vi "Compass on GIC parallel 2.vi"(11 "GIC Input 2":T1={"     Use ?\nOff       On"=[FALSE, TRUE, FALSE, TRUE], "Mode:"=FALSE, "Extra Port"="", "Hokuyo Port"="COM7", "Tx Prop  Port"="COM6", "Compass Port"="", "GPS Port"="", "Num of WPs"=0, "WP Lats and Longs"={"WP Lats"=[], "WP Longs"=[]}, "Obst Lats and Longs"={"Obst Lats"=[], "Obst Longs"=[]}, "Parameters"=[], "GPS Data"=[], "Compass"=0.0, "LMS Vector"=[], "Vision Vector"=[], "Direction Cmd"=0.0, "Speed Cmd"=0.0, "WP Vector"=[], "WP Number"=0, "Extra"=0, "SW Map"=[], "Path Cluster"={"Path x node"=[], "Path y node"=[]}, "Sim Course"=[]} {"Obst Lats and Longs"."Obst Longs" format="%#_8g"; "Obst Lats and Longs"."Obst Lats" format="%#_8g"}) -> ()   [LabVIEW 2014]
uses:
  Global_vars.vi
panel:
  out "compass out":dbl
  # "Compass on GIC parallel 2"
  # "Compass on New GIC A"
  # "Input:"
  # "Output:"
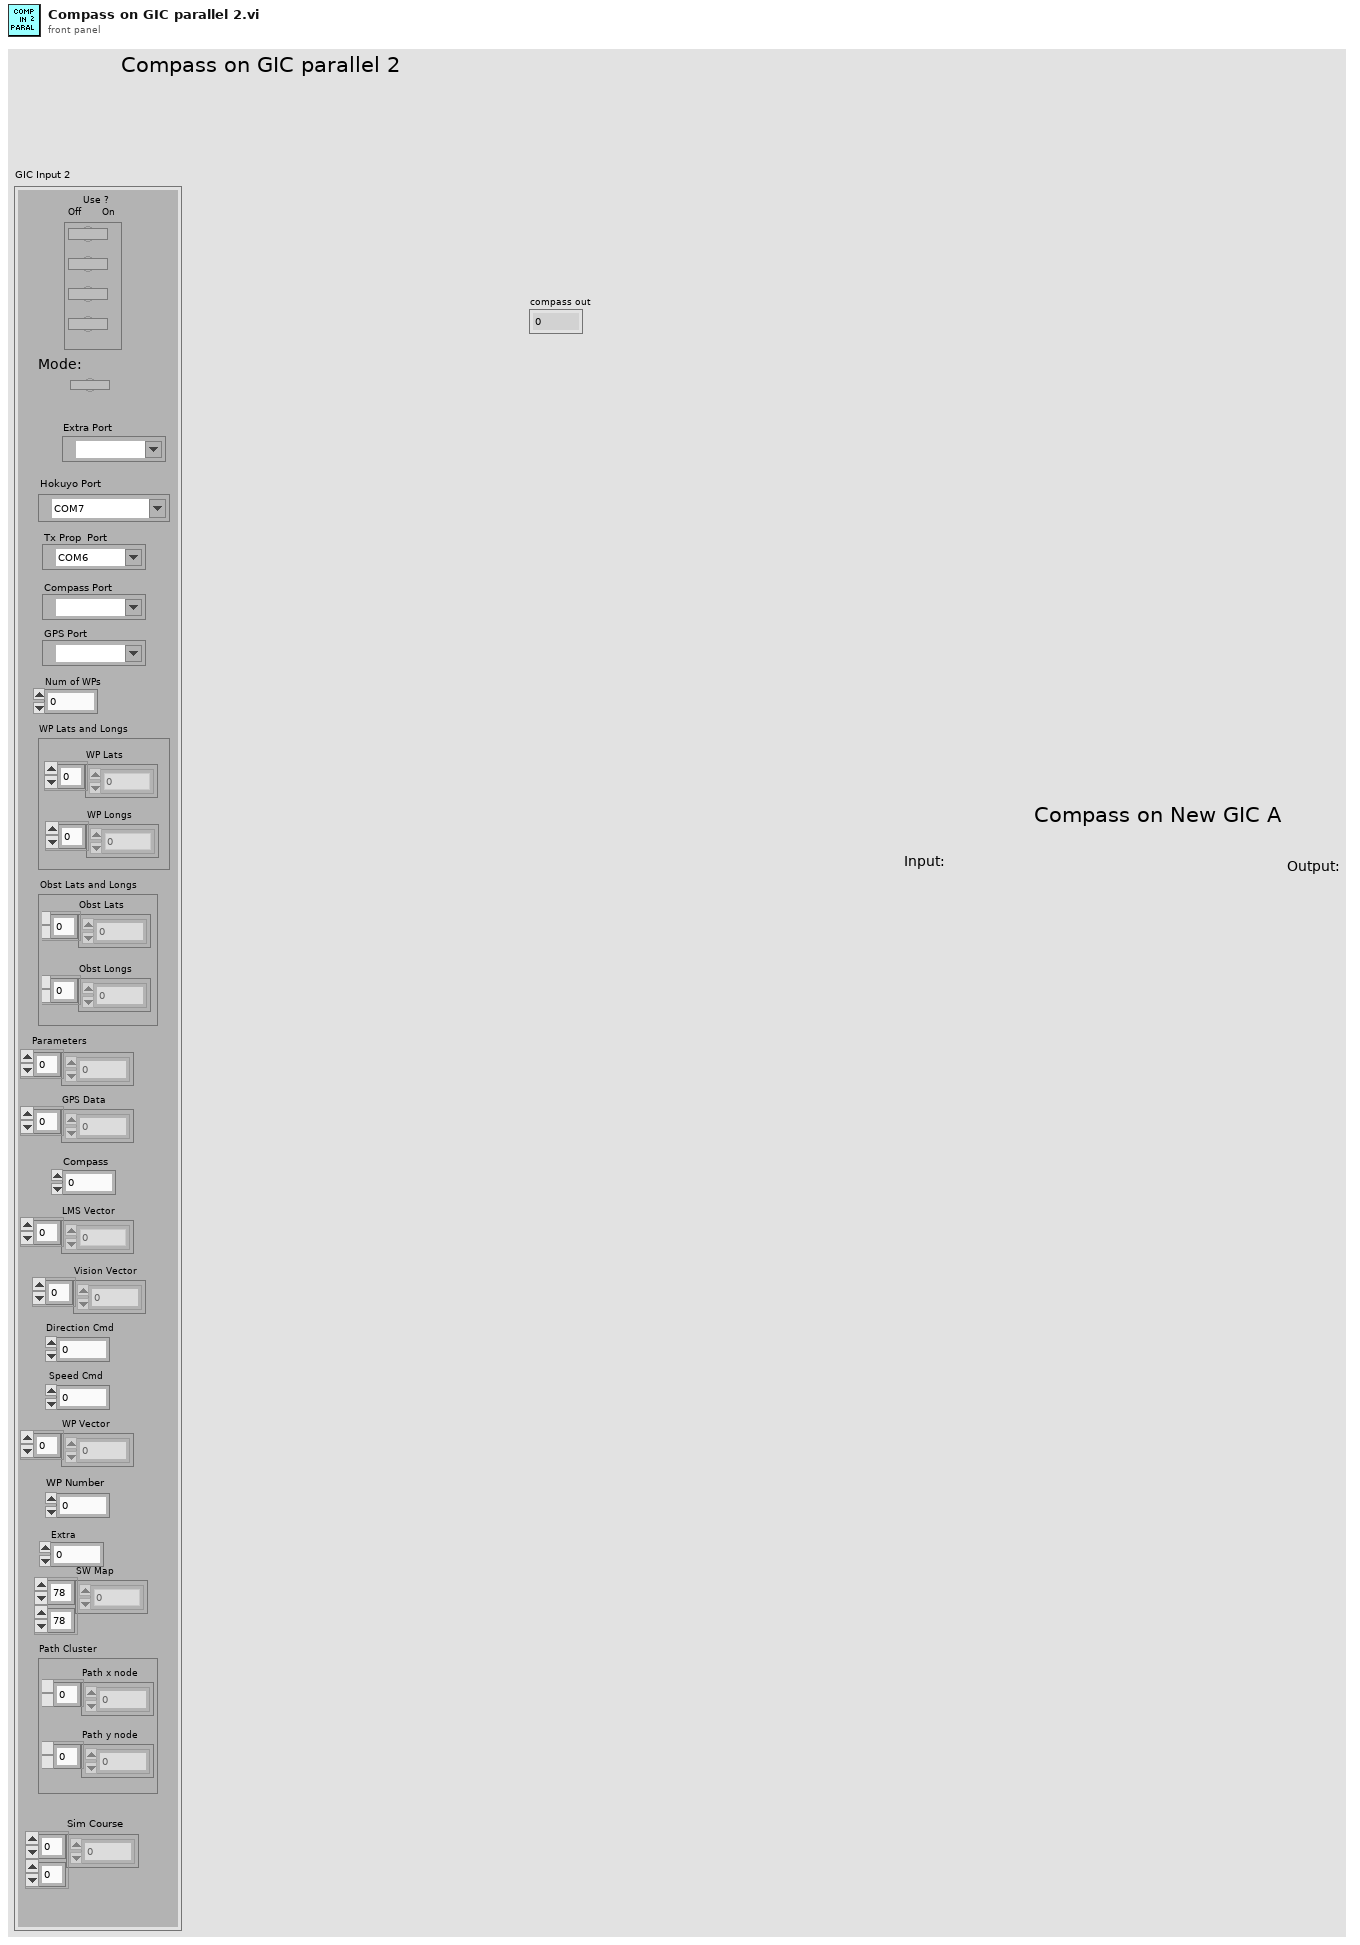
[diagram p1: front panel]
types:
  T1 = cluster{"     Use ?\nOff       On":bool[], "Mode:":bool, "Extra Port":refnum<visa-resource-name>, "Hokuyo Port":refnum<visa-resource-name>, "Tx Prop  Port":refnum<visa-resource-name>, "Compass Port":refnum<visa-resource-name>, "GPS Port":refnum<visa-resource-name>, "Num of WPs":i16, "WP Lats and Longs":cluster{"WP Lats":dbl[], "WP Longs":dbl[]}, "Obst Lats and Longs":cluster{"Obst Lats":dbl[], "Obst Longs":dbl[]}, "Parameters":dbl[], "GPS Data":dbl[], "Compass":dbl, "LMS Vector":dbl[], "Vision Vector":dbl[], "Direction Cmd":dbl, "Speed Cmd":dbl, "WP Vector":dbl[], "WP Number":i32, "Extra":i16, "SW Map":i32[][], "Path Cluster":cluster{"Path x node":dbl[], "Path y node":dbl[]}, "Sim Course":i8[][]}
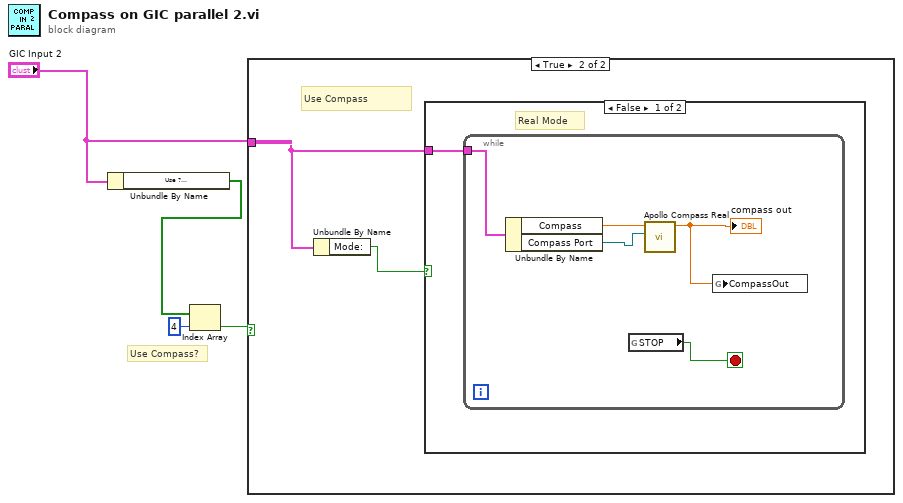
[diagram p0: block diagram]
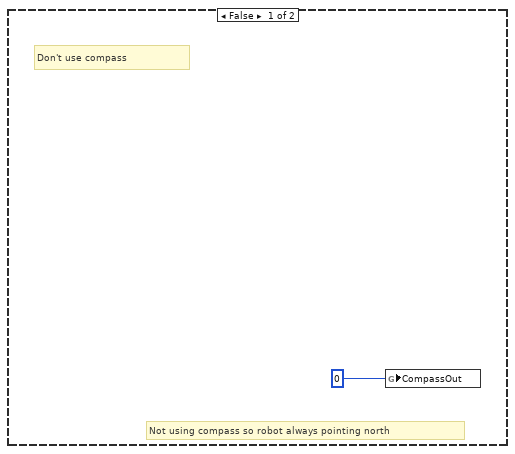
[diagram p2: hidden frame]
diagram:
  # "Use Compass?"
  n1 = Unbundle By Name("GIC Input 2") -> ("Use ?\nOff       On"=w4:bool[])
  n2 = Index Array(array=w4, index=4) -> (element=w2:bool)
  n3 = case shown="True" w2 {
    tunnel: "GIC Input 2" -> [_ w7]
    frame False {
      # "Don't use compass"
      # "Not using compass so robot always pointing north"
      n4 = global write "Global_vars.vi" "CompassOut"(0) -> ()
    }
    frame True {
      # "Use Compass"
      n5 = Unbundle By Name(w7) -> ("Mode:"=w6:bool)
      n6 = case shown="False" w6 {
        tunnel: w7 -> [w8 _]
        frame False {
          # "Real Mode"
          n7 = while {
            tunnel: w8 -> [w12]
            stop <- w9 stop-if-true
            n8 = Unbundle By Name(w12) -> ("Compass"=w10:dbl, "Compass Port"=w13:refnum<visa-resource-name>)
            n9 = global read "Global_vars.vi" "STOP"() -> (w9:bool)
            n10 = call "Apollo Compass Real.vi"("Compass Com Port"=w13, "Compass In"=w10) -> ("Compass Out"=w11:dbl)  [unwired: 8 in]
            "compass out" <- w11
            n11 = global write "Global_vars.vi" "CompassOut"(w11) -> ()
          }
        }
        frame True {
          # "This mode done in main flat sequence"
          # "Simulation mode"
        }
      }
    }
  }
